vi "Test Get Default Value for Type.vi"(8 "error in":errorcluster, 10 "types to test":variant[](array[variant])) -> (0 "error out":errorcluster, 2 "passed":bool)   [LabVIEW 2020, in "test_openg_variant.lvlib"]
uses:
  test_openg_variant.lvlib
  source/library/openg_variant.lvlib
  <vilib>/addons/_JKI Toolkits/Caraya/classes/Assert/Assert.lvclass
  <vilib>/addons/_JKI Toolkits/Caraya/classes/Test/Test.lvclass
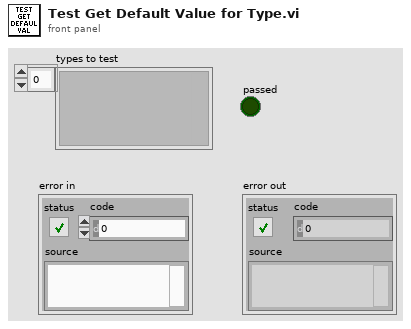
[diagram p1: front panel]
types:
  T1 = typedef "openg_variant.lvlib/Type Descriptor Header.ctl" = cluster{"length":u16, "private":u8, "type":T2, "# elements":u16}
  T2 = typedef "openg_variant.lvlib/Type Descriptor Enumeration.ctl" = enum8{"<Null>", "I8", "I16", "I32", "I64", "U8", "U16", "U32", "U64", "SGL", "DBL", "EXT", "CSG", "CDB", "CXT", "0x0F", "0x10", "0x11", "0x12", "0x13", "0x14", "Enum U8", "Enum U16", "Enum U32", "Enum U64", "SGL PQ", "DBL PQ", "EXT PQ", "CSG PQ", "CDB PQ", "CXT PQ", "0x1F", "0x20", "Boolean", "0x22", "0x23", "0x24", "0x25", "0x26", "0x27", "0x28", "0x29", "0x2A", "0x2B", "0x2C", "0x2D", "0x2E", "0x2F", "String", "0x31", "Path", "Pict", "0x34", "0x35", "0x36", "DAQ", "0x38", "0x39", "0x3A", "0x3B", "0x3C", "0x3D", "0x3E", "0x3F", "Array", "0x41", "0x42", "0x43", "0x44", "0x45", "0x46", "0x47", "0x48", "0x49", "0x4A", "0x4B", "0x4C", "0x4D", "0x4E", "0x4F", "Cluster", "0x51", "0x52", "Variant", "Waveform", "0x55", "0x56", "0x57", "0x58", "0x59", "0x5A", "0x5B", "0x5C", "0x5D", "0x5E", "Fixed Point", "0x60", "0x61", "0x62", "0x63", "0x64", "0x65", "0x66", "0x67", "0x68", "0x69", "0x6A", "0x6B", "0x6C", "0x6D", "0x6E", "0x6F", "Refnum", "0x71", "0x72", "Set Collection", "Map Collection"}
  T3 = typedef "openg_variant.lvlib/Type Descriptor.ctl" = i16[]
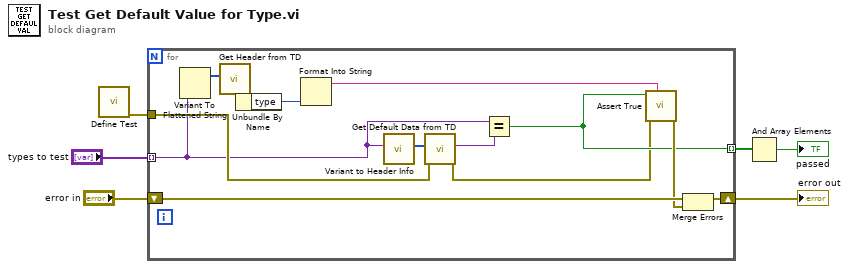
[diagram p0: block diagram]
diagram:
  n1 = call <vilib>:"Define Test.vi"() -> ("error out"=w6:errorcluster)  [unwired: 10 in, 1 out]
  n2 = for {
    tunnel: "types to test" -> [w9] mode=indexing
    shift-right: [w17] -> w3
    shift-left: "error in" -> [w19]
    tunnel: [w8] -> w5 mode=indexing
    tunnel: w6 -> [w10]
    n3 = Variant To Flattened String(Variant=w9) -> (1:w16:i16[])  [unwired: 1 out]
    n4 = call "Get Header from TD.vi"("Type Descriptor"=w16) -> ("Type Descriptor Header"=w15:T1)
    n5 = Unbundle By Name(w15) -> ("type"=w14:T2)
    n6 = Format Into String(w14) -> (resulting string=w13:string)  [unwired: 3 in, 1 out]
    n7 = call "Variant to Header Info.vi"("Variant"=w9) -> ("Type Descriptor"=w11:T3)  [unwired: 3 in, 2 out]
    n8 = call "Get Default Data from TD.vi"("error in (no error)"=w10, "Type Descriptor"=w11) -> ("error out"=w7:errorcluster, "Default VData"=w12:variant)  [unwired: 8 in]
    n9 = Equal?(x=w9, y=w12) -> (x = y?=w8:bool)
    n10 = call <vilib>:"Assert True.vi"("Label"=w13, "error in (no error)"=w7, "True?"=w8) -> ("error out"=w18:errorcluster)  [unwired: 7 in, 1 out]
    n11 = Merge Errors(w19, w18) -> (w17:errorcluster)
  }
  "error out" <- w3
  n12 = And Array Elements(Boolean array=w5) -> (logical AND=→"passed":bool)
